vi "Functional Imaging-Select image.vi"(8 "error in (no error)":errorcluster) -> (0 "error out":errorcluster, 3 "SelectedPOIMax":T1)   [LabVIEW 2013]
uses:
  <vilib>/vision/Image Controls.llb/IMAQ Image.ctl
  Typedefs/Overlay FG functions.ctl
  Global variables/gl_Functional Imaging-Global variables.vi
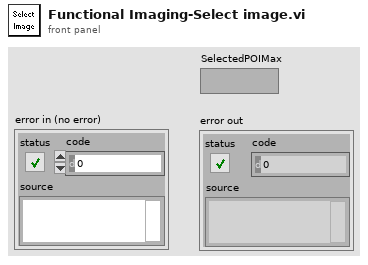
[diagram p1: front panel]
types:
  T1 = typedef "IMAQ Image.ctl" = refnum<image>
  T2 = typedef "Overlay FG functions.ctl" = enum16{"Generate new images", "Get stored images", "Clear"}
  T3 = typedef "Functional Imging UI Refs.ctl" = cluster{"Menu ref":refnum<k9>, "Image control":refnum<vi>, "VI ref":refnum<vi>, "XGrapher":refnum<vi>, "Smoothing":refnum<vi>, "POI Averaging":refnum<vi>, "Normalize":refnum<vi>, "POI data points in each trial":refnum<vi>, "Channel":refnum<vi>, "Experiment data folder path":refnum<vi>, "[ROI vis]":refnum<vi>, "[Groups] visbl":T4, "Group Name":refnum<vi>, "POI index":refnum<vi>, "Trial No.":refnum<vi>, "Intensity Zoom":refnum<vi>, "Trial Cursor Enabled":refnum<vi>, "Number of Trials (ind 1)":refnum<vi>, "Number of Trials (ind 2)":refnum<vi>, "MiniScans Available":refnum<vi>, "POI Available":refnum<vi>, "Defer graph updates":refnum<vi>, "Waveform selector":refnum<vi>, "#of selected POI":refnum<vi>, "#of selected MiniScans":refnum<vi>, "#of selected groups":refnum<vi>, "Max Z-Projection":refnum<vi>, "Z-Plane Selector":refnum<vi>, "Index of miniscan point to visualise":refnum<vi>, "ROI vis. mode":refnum<vi>, "Total # of points":refnum<vi>, "Index of group clicked on":refnum<vi>, "Pane 1":refnum<vi>, "Pane 2":refnum<vi>, "Pane 3":refnum<vi>, "Pane 4":refnum<vi>, "Pane 5":refnum<vi>, "Pane 6":refnum<vi>, "Deselect all ROI":refnum<vi>, "Deselect all groups":refnum<vi>}
  T4 = typedef "Groups array referecne.ctl" = refnum<vi>
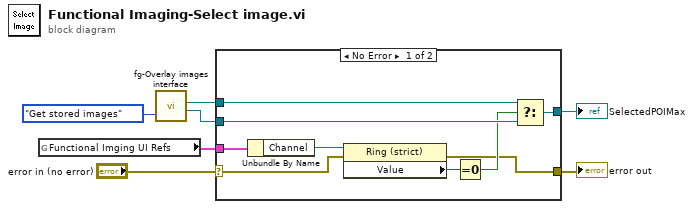
[diagram p0: block diagram]
diagram:
  n1 = global read "gl_Functional Imaging-Global variables.vi" "Functional Imging UI Refs"() -> (w1:T3)
  n2 = call "fg-Overlay images interface.vi"("Function"=Overlay_FG_functions."Get stored images") -> ("GreenPOIMax"=w3:T1, "RedPOIMax"=w4:T1)  [unwired: 8 in, 1 out]
  n3 = case shown="No Error" "error in (no error)" {
    selector: "error in (no error)" -> [w9 w17]
    tunnel: w3 -> [w16 _]
    tunnel: w4 -> [w15 _]
    tunnel: w1 -> [w12 _]
    tunnel: [w10 _] -> w7
    tunnel: [w8 w17] -> w5
    frame No Error {
      n4 = Unbundle By Name(w12) -> ("Channel"=w13:refnum<vi>)
      n5 = property class="Ring (strict)"(reference=w13, error in=w9) -> (error out=w8:errorcluster, "Value"=w14:u16)  [unwired: 1 out]
      n6 = Equal To 0?(x=w14) -> (x = 0?=w11:bool)
      n7 = Select(t=w15, s=w11, f=w16) -> (s? t:f=w10:T1)
    }
    frame Error {
    }
  }
  "SelectedPOIMax" <- w7
  "error out" <- w5
